vi "Gcode loader.vi"(4 "Stop":refnum<vi>, 5 "3D Graph":refnum<vi>, 6 "Fast load":bool, 7 "XYGraph in":refnum<vi>, 8 "error in (no error)":errorcluster, 11 "Data cluster":T1) -> (0 "error out":errorcluster, 3 "Data cluster out":T1)   [LabVIEW 2020]
uses:
  <vilib>/Native 3D Graph/xcontrol/3DPC_SurfacePlot.xctl
  controls/Pattern recognizer data.ctl
  <vilib>/Native 3D Graph/classes/Base Datatype.lvclass
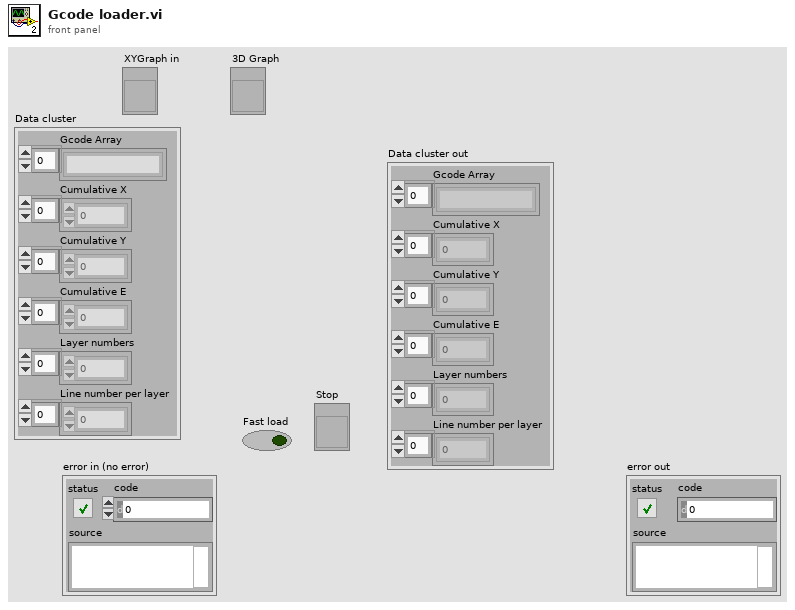
[diagram p1: front panel]
types:
  T1 = typedef "Pattern recognizer data.ctl" = cluster{"Gcode Array":string[], "Cumulative X":dbl[], "Cumulative Y":dbl[], "Cumulative E":dbl[], "Layer numbers":i32[], "Line number per layer":i32[]}
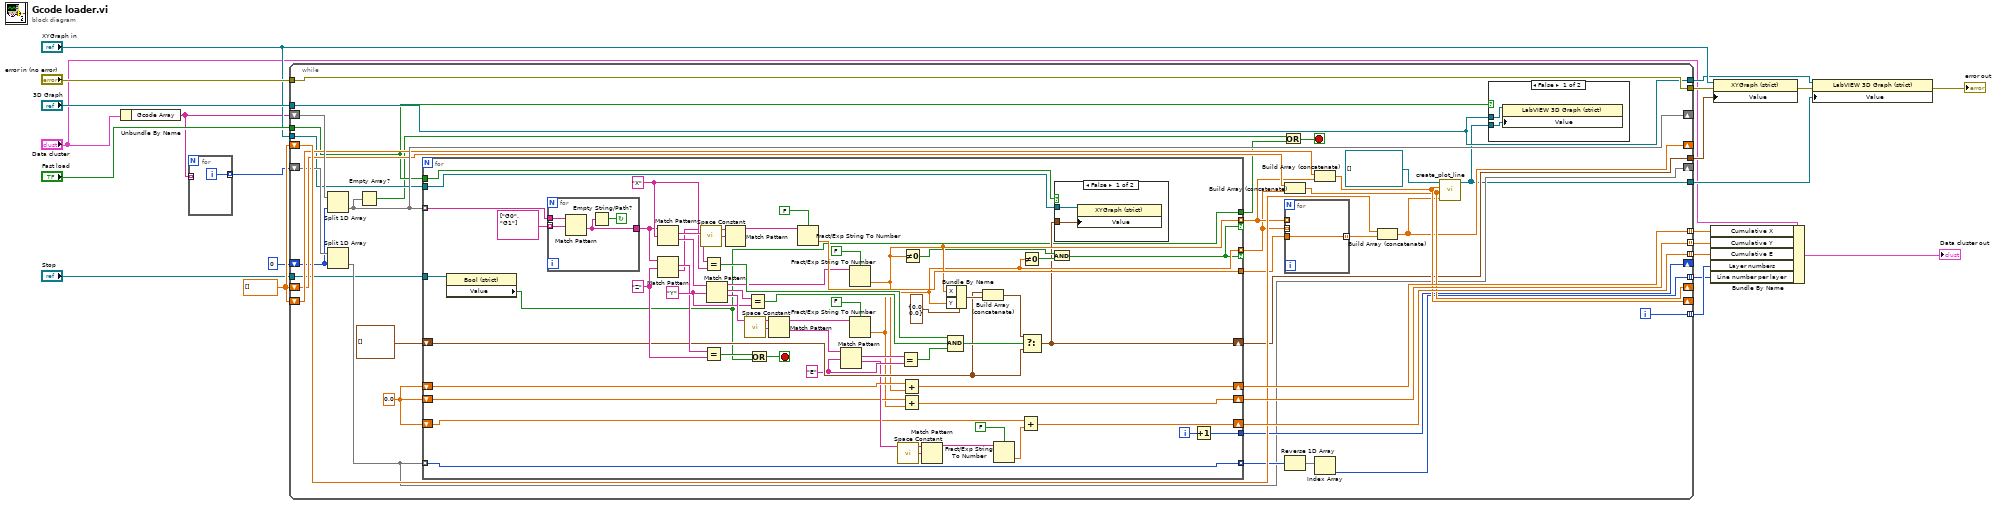
[diagram p0: block diagram]
diagram:
  w20 = dbl[] []
  n1 = Unbundle By Name("Data cluster") -> ("Gcode Array"=w3:string[])
  n2 = for {
    tunnel: [w23] -> w10 mode=indexing
    tunnel: w3 -> [_] mode=indexing
    i -> [w23]
  }
  n3 = while {
    shift-right: [w40] -> _
    shift-left: 0 -> [w36]
    shift-right: [w59] -> _
    shift-left: w3 -> [w56]
    tunnel: [w57] -> w9 mode=indexing
    tunnel: [w54] -> w8 mode=indexing
    tunnel: [w53] -> w7 mode=indexing
    shift-right: [w46] -> _
    shift-left: w20 -> [w51]
    shift-right: [w48] -> _
    shift-left: w20 -> [w50]
    shift-right: [w47] -> _
    shift-left: w20 -> [w49]
    tunnel: [w41] -> w5 mode=indexing
    tunnel: [w35] -> w4 mode=indexing
    shift-right: [w34] -> _
    shift-left: w10 -> [w37]
    tunnel: [w33] -> w16
    tunnel: "error in (no error)" -> [w33]
    tunnel: "XYGraph in" -> [w32]
    tunnel: "3D Graph" -> [w30]
    tunnel: "Fast load" -> [w28]
    tunnel: [w31] -> w15
    tunnel: [w30] -> w13
    tunnel: [w29] -> w11
    tunnel: "Stop" -> [w27]
    i -> [w41]
    stop <- w24 stop-if-true
    w55 = 0.0
    n4 = Split 1D Array(array=w56, index=w36) -> (second subarray=w59:string[])  [unwired: 1 out]
    n5 = Split 1D Array(array=w37, index=w36) -> (second subarray=w34:i32[])  [unwired: 1 out]
    n6 = Empty Array?(array=w59) -> (empty?=w25:bool)
    n7 = for {
      tunnel: w59 -> [w120] mode=indexing
      tunnel: [w72] -> w40
      shift-right: [w70] -> w31
      shift-left: cluster{"X":dbl, "Y":dbl}[] [] ("XY Graph 2") -> [w100]
      shift-right: [w94] -> w57
      shift-left: w55 -> [w95]
      shift-right: [w88] -> w54
      shift-left: w55 -> [w90]
      shift-right: [w86] -> w53
      shift-left: w55 -> [w89]
      tunnel: [w78] -> w42
      tunnel: [w77] -> w45 mode=indexing if=w73
      tunnel: [w76] -> w44 mode=indexing if=w73
      tunnel: [w71] -> w39 mode=indexing
      tunnel: w34 -> [w71] mode=indexing
      tunnel: w32 -> [w69]
      tunnel: w28 -> [w68]
      tunnel: w27 -> [w66]
      tunnel: [w63] -> w26
      i -> [w104]
      stop <- w64 stop-if-true
      w98 = "E" ("regular expression")
      w105 = "Z" ("regular expression")
      w112 = "Y" ("regular expression")
      w114 = "X" ("regular expression")
      n8 = property on="Property Node" class="Bool (strict)"(reference=w66) -> ("Value"=w63:bool)  [unwired: 1 in, 2 out]
      n9 = for {
        tunnel: string[] ["G0", "G1"] ("regular expression") -> [w125] mode=indexing
        tunnel: w120 -> [w126]
        tunnel: [w124] -> w107
        stop <- w123 continue-if-true
        n10 = Match Pattern(string=w126, regular expression=w125) -> (after substring=w124:string)  [unwired: 1 in, 3 out]
        n11 = Empty String/Path?(string/path=w124) -> (empty?=w123:bool)
      }
      n12 = Match Pattern(string=w107, regular expression=w114) -> (match substring=w115:string, after substring=w118:string)  [unwired: 1 in, 2 out]
      n13 = Match Pattern(string=w107, regular expression=w105) -> (match substring=w106:string, after substring=w80:string)  [unwired: 1 in, 2 out]
      n14 = call <vilib>:"Space Constant.vi"() -> ("String"=w82:string)
      n15 = Equal?(x=w115, y=w114) -> (x = y?=w111:bool)
      n16 = Equal?(x=w106, y=w105) -> (x = y?=w65:bool)
      n17 = Match Pattern(string=w118, regular expression=w112) -> (before substring=w67:string, match substring=w113:string, after substring=w117:string)  [unwired: 1 in, 1 out]
      n18 = Match Pattern(string=w80, regular expression=w82) -> (before substring=w81:string)  [unwired: 1 in, 3 out]
      n19 = call <vilib>:"Space Constant.vi"() -> ("String"=w116:string)
      n20 = Equal?(x=w113, y=w112) -> (x = y?=w110:bool)
      n21 = Or(x=w65, y=w63) -> (x .or. y?=w64:bool)
      n22 = Match Pattern(string=w117, regular expression=w116) -> (before substring=w109:string, after substring=w97:string)  [unwired: 1 in, 2 out]
      n23 = Fract/Exp String To Number(use system decimal point (T)=FALSE, string=w81) -> (number=w78:dbl)  [unwired: 2 in, 1 out]
      n24 = Match Pattern(string=w97, regular expression=w98) -> (match substring=w99:string, after substring=w92:string)  [unwired: 1 in, 2 out]
      n25 = Fract/Exp String To Number(use system decimal point (T)=FALSE, string=w67) -> (number=w77:dbl)  [unwired: 2 in, 1 out]
      n26 = Fract/Exp String To Number(use system decimal point (T)=FALSE, string=w109) -> (number=w76:dbl)  [unwired: 2 in, 1 out]
      n27 = call <vilib>:"Space Constant.vi"() -> ("String"=w93:string)
      n28 = Equal?(x=w99, y=w98) -> (x = y?=w96:bool)
      n29 = Add(x=w95, y=w77) -> (x+y=w94:dbl)
      n30 = Add(x=w90, y=w76) -> (x+y=w88:dbl)
      n31 = Not Equal To 0?(x=w77) -> (x != 0?=w75:bool)
      n32 = Match Pattern(string=w92, regular expression=w93) -> (before substring=w91:string)  [unwired: 1 in, 3 out]
      n33 = Bundle By Name(cluster=cluster{"X":dbl, "Y":dbl} {"X"=0.0, "Y"=0.0} ("XY Graph"), "X"=w77, "Y"=w76) -> (w101:cluster{"X":dbl, "Y":dbl})
      n34 = Compound Arithmetic op=AND(w111, w110, w96) -> (w103:bool)
      n35 = Build Array (concatenate)(w100, w101) -> (w102:cluster{"X":dbl, "Y":dbl}[])
      n36 = Fract/Exp String To Number(use system decimal point (T)=FALSE, string=w91) -> (number=w87:dbl)  [unwired: 2 in, 1 out]
      n37 = Add(x=w89, y=w87) -> (x+y=w86:dbl)
      n38 = Not Equal To 0?(x=w76) -> (x != 0?=w74:bool)
      n39 = Select(t=w102, s=w103, f=w100) -> (s? t:f=w70:cluster{"X":dbl, "Y":dbl}[])
      n40 = And(x=w75, y=w74) -> (x .and. y?=w73:bool)
      n41 = case shown="False" w68 {
        tunnel: w70 -> [w122 _]
        tunnel: w69 -> [w121 _]
        frame False {
          n42 = property class="XYGraph (strict)"(reference=w121, "Value"=w122) -> ()  [unwired: 1 in, 2 out]
        }
        frame True {
        }
      }
      n43 = Increment(x=w104) -> (x+1=w72:i32)
    }
    n44 = Or(x=w25, y=w26) -> (x .or. y?=w24:bool)
    n45 = Build Array (concatenate)(w49, w44) -> (w47:dbl[])
    n46 = for {
      tunnel: [w62] -> w52 mode=indexing
      tunnel: w42 -> [w62]
      tunnel: w45 -> [_] mode=indexing
      tunnel: w44 -> [_] mode=indexing
    }
    n47 = Reverse 1D Array(array=w39) -> (reversed array=w38:i32[])
    n48 = Build Array (concatenate)(w50, w45) -> (w48:dbl[])
    n49 = Index Array(array=w38) -> (element=w35:i32)  [unwired: 1 in]
    n50 = Build Array (concatenate)(w51, w52) -> (w46:dbl[])
    n51 = call <vilib>:"create_plot_line.vi"("z vector"=w46, "y vector"=w47, "x vector"=w48, "plots in"=refnum<class "Base Datatype.lvclass">[] []) -> ("plots out"=w29:refnum<class "Base Datatype.lvclass">[])  [unwired: 1 in, 6 out]
    n52 = case shown="False" w28 {
      tunnel: w29 -> [w61 _]
      tunnel: w30 -> [w60 _]
      frame False {
        n53 = property class="LabVIEW 3D Graph (strict)"(reference=w60, "Value"=w61) -> ()  [unwired: 1 in, 2 out]
      }
      frame True {
      }
    }
  }
  n54 = Bundle By Name(cluster="Data cluster", "Cumulative X"=w9, "Cumulative Y"=w8, "Cumulative E"=w7, "Layer numbers"=w5, "Line number per layer"=w4) -> (→"Data cluster out":T1)
  n55 = property class="XYGraph (strict)"(reference="XYGraph in", error in=w16, "Value"=w15) -> (error out=w14:errorcluster)  [unwired: 1 out]
  n56 = property class="LabVIEW 3D Graph (strict)"(reference=w13, error in=w14, "Value"=w11) -> (error out=→"error out":errorcluster)  [unwired: 1 out]
